vi "Check VISA Inst Type.vi"(3 "Error In":errorcluster, 4 "Check Parameters":T1={"Instrument"="Instrument", "ID Test String"="", "Terminator Character"="", "wait (mS)"=0, "Wait For SRQ"=FALSE}, 5 "VISA session":refnum<visa-resource-name>) -> (0 "Error Out":errorcluster, 1 "ID":string, 2 "dup VISA session":refnum<visa-resource-name>)   [LabVIEW 2024]
doc: "This VI checks that an instrument is of the expected type at a given GPIB bus address.\nScott Hannahs, <sth@magnet.fsu.edu> NHMFL-FSU, May 2003"
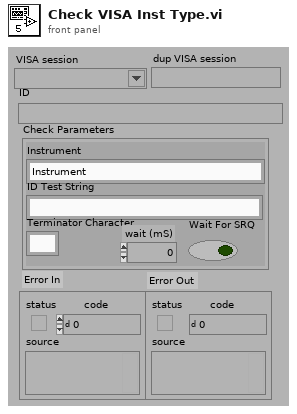
[diagram p1: front panel]
types:
  T1 = cluster{"Instrument":string, "ID Test String":string, "Terminator Character":string, "wait (mS)":u32, "Wait For SRQ":bool}
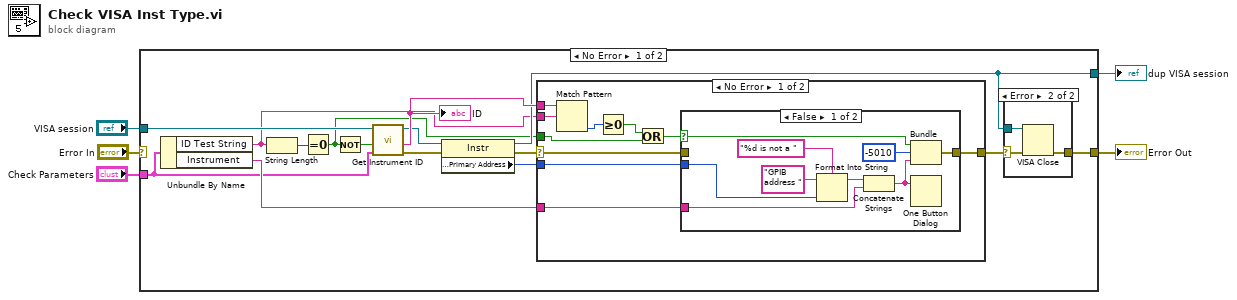
[diagram p0: block diagram]
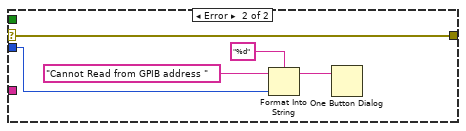
[diagram p4: hidden frame]
diagram:
  n1 = case shown="No Error" "Error In" {
    selector: "Error In" -> [_ w50]
    tunnel: [w14 w50] -> w5
    tunnel: "VISA session" -> [w12 w51]
    tunnel: [w13 w51] -> w2
    tunnel: "Check Parameters" -> [w7 _]
    frame No Error {
      n2 = Unbundle By Name(w7) -> ("ID Test String"=w6:string, "Instrument"=w20:string)
      n3 = String Length(string=w6) -> (length=w10:i32)
      n4 = Equal To 0?(x=w10) -> (x = 0?=w8:bool)
      n5 = Not(x=w8) -> (.not. x?=w9:bool)
      n6 = call "Get Instrument ID.vi"("Check Parameters"=w7, "Check ID"=w9, "VISA resource name"=w12) -> ("Error Out"=w18:errorcluster, "Instrument ID"=w19:string, "VISA resource name"=w17:refnum<visa-resource-name>)  [unwired: 2 in]
      "ID" <- w19
      n7 = property class="Instr"(reference=w17, error in=w18) -> (reference out=w13:refnum<visa-resource-name>, error out=w11:errorcluster, "GPIB Settings:Primary Address"=w16:u16)
      n8 = case shown="No Error" w11 {
        selector: w11 -> [w25 w45]
        tunnel: [w31 w45] -> w15
        tunnel: w6 -> [w34 _]
        tunnel: w19 -> [w32 _]
        tunnel: w20 -> [w30 _]
        tunnel: w16 -> [w29 w46]
        tunnel: w8 -> [w26 _]
        frame No Error {
          n9 = Match Pattern(string=w32, regular expression=w34) -> (offset past match=w33:i32)  [unwired: 1 in, 3 out]
          n10 = Greater Or Equal To 0?(x=w33) -> (x >= 0?=w27:bool)
          n11 = Or(x=w27, y=w26) -> (x .or. y?=w28:bool)
          n12 = case shown="False" w28 {
            selector: w28 -> [w39 _]
            tunnel: [w40 w44] -> w31
            tunnel: w30 -> [w36 _]
            tunnel: w29 -> [w35 _]
            tunnel: w25 -> [_ w44]
            frame False {
              n13 = Format Into String(format string="%d is not a ", initial string="GPIB address ", w35) -> (resulting string=w43:string)  [unwired: 1 in, 1 out]
              n14 = Concatenate Strings(w43, w36) -> (w37:string)
              n15 = Bundle(w39, -5010, w37) -> (w40:errorcluster)  [unwired: 1 in]
              n16 = One Button Dialog(message=w37) -> ()  [unwired: 1 in, 1 out]
            }
            frame True {
            }
          }
        }
        frame Error {
          n17 = Format Into String(format string="%d", initial string="Cannot Read from GPIB address ", w46) -> (resulting string=w47:string)  [unwired: 1 in, 1 out]
          n18 = One Button Dialog(message=w47) -> ()  [unwired: 1 in, 1 out]
        }
      }
      n19 = case shown="Error" w15 {
        selector: w15 -> [w21 w22]
        tunnel: [w21 w24] -> w14
        tunnel: w13 -> [_ w23]
        frame No Error {
        }
        frame Error {
          n20 = VISA Close(VISA resource name=w23, error in (no error)=w22) -> (error out=w24:errorcluster)
        }
      }
    }
    frame Error {
    }
  }
  "Error Out" <- w5
  "dup VISA session" <- w2
